vi "Test Matrix Subtract.vi"() -> ()   [LabVIEW 2014, in "Arduino MatrixMath.lvlib"]
uses:
  Arduino MatrixMath.lvlib
panel:
  out "Error Out":errorcluster
  in  "Error In":errorcluster
  in  "B":sgl[](array[numeric])=[1.0, 2.0, 3.0, 4.0, 5.0, 6.0, 7.0, 8.0]
  out "C":sgl[](array[numeric])
  in  "A":sgl[](array[numeric])=[1.0, 2.0, 3.0, 4.0, 5.0, 6.0, 7.0, 8.0]
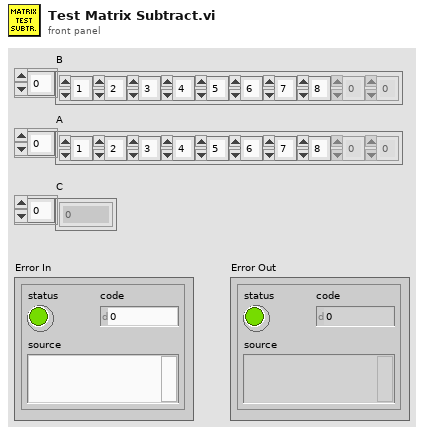
[diagram p1: front panel]
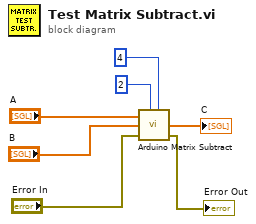
[diagram p0: block diagram]
diagram:
  n1 = call "Arduino Matrix Subtract.vi"("A"="A", "rows num."=u8 2, "B"="B", "Error In"="Error In", "cols num."=u8 4) -> ("A-B"=→"C":sgl[], "Error Out"=→"Error Out":errorcluster)  [unwired: 3 in]
